vi "Meas Result Get Sweep Data.vi"(3 "freq filter (NaN: no filter)":dbl=nan, 4 "uncertainty mode":T1, 5 "phase index (default: 0)":i32, 6 "result":T4) -> (0 "quantities":T2, 1 "unc(data)":T3, 2 "data":T3)   [LabVIEW 2013]
doc: "Processes collected readings into sweep with uncertainties in selected mode."
uses:
  Meas Results Sweep Data.ctl
  Meas Results.ctl
  bridge/Bridge Frequency Readings Data.ctl
  drivers/TWM client/Meas Proc QWTB Spectrum Data.ctl
  Meas Quantity Names.ctl
  Meas Results Sweep Data Uncertainty Mode.ctl
  varilib/varilib.lvlib
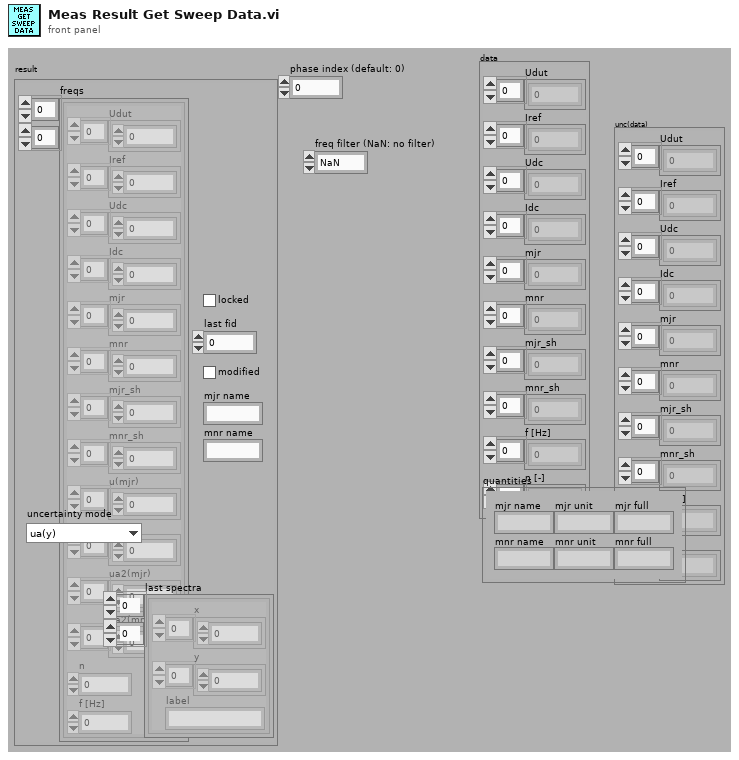
[diagram p1: front panel]
types:
  T1 = typedef "Meas Results Sweep Data Uncertainty Mode.ctl" = enum16{"ua(y)", "ua(y) (p=95%)", "uc(y) (p=95%)"}
  T2 = typedef "Meas Quantity Names.ctl" = cluster{"mjr name":string, "mnr name":string, "mjr unit":string, "mnr unit":string, "mjr full":string, "mnr full":string}
  T3 = typedef "Meas Results Sweep Data.ctl" = cluster{"Udut":dbl[], "Iref":dbl[], "Udc":dbl[], "Idc":dbl[], "mjr":dbl[], "mnr":dbl[], "mjr_sh":dbl[], "mnr_sh":dbl[], "f [Hz]":dbl[], "n [-]":i32[]}
  T4 = typedef "Meas Results.ctl" = cluster{"freqs":T5[][], "locked":bool, "last fid":i32, "modified":bool, "mjr name":string, "mnr name":string, "last spectra":T6[][]}
  T5 = typedef "Bridge Frequency Readings Data.ctl" = cluster{"Udut":dbl[], "Iref":dbl[], "Udc":dbl[], "Idc":dbl[], "mjr":dbl[], "mnr":dbl[], "mjr_sh":dbl[], "mnr_sh":dbl[], "u(mjr)":dbl[], "u(mnr)":dbl[], "ua2(mjr)":dbl[], "ua2(mnr)":dbl[], "n":i32, "f [Hz]":dbl}
  T6 = typedef "Meas Proc QWTB Spectrum Data.ctl" = cluster{"x":sgl[], "y":sgl[], "label":string}
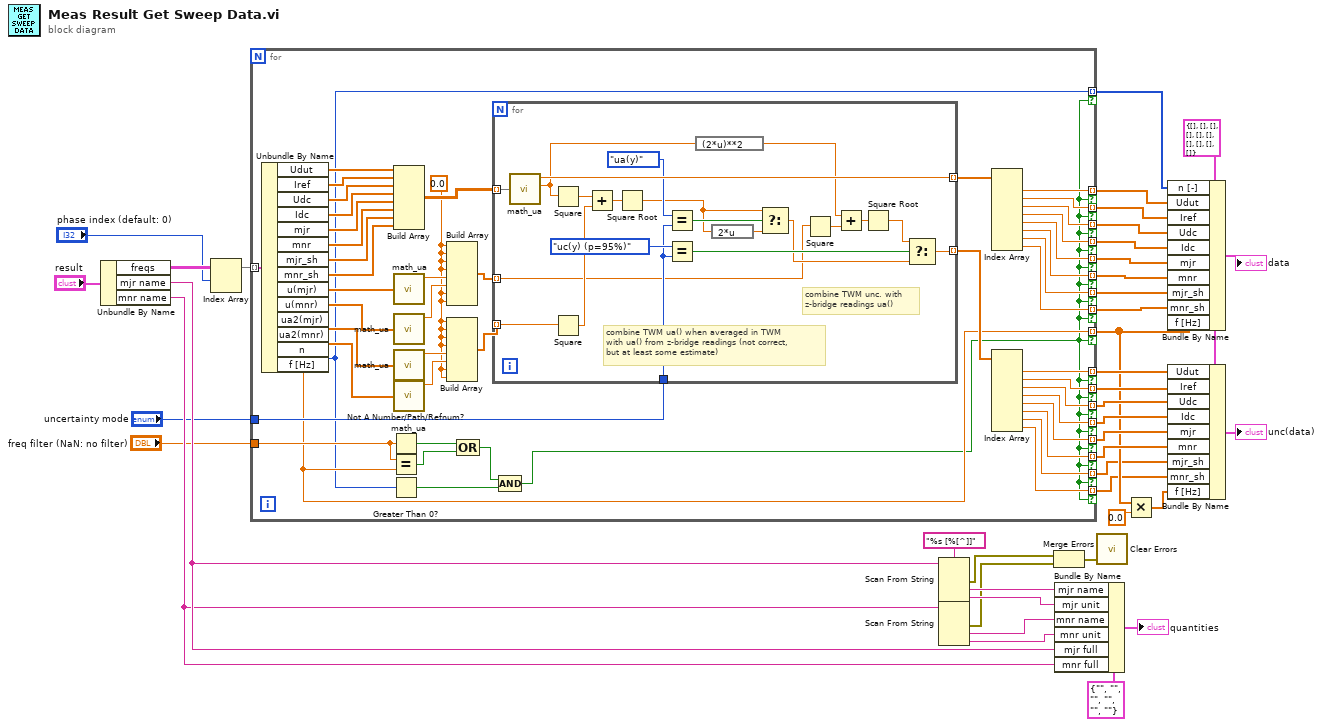
[diagram p0: block diagram]
diagram:
  w18 = "%s [%[^]]" ("format string")
  w24 = T3 {"Udut"=[], "Iref"=[], "Udc"=[], "Idc"=[], "mjr"=[], "mnr"=[], "mjr_sh"=[], "mnr_sh"=[], "f [Hz]"=[], "n [-]"=[]} ("data")
  n1 = Unbundle By Name("result") -> ("freqs"=w40:T5[][], "mjr name"=w15:string, "mnr name"=w14:string)
  n2 = Index Array(array=w40, index (row)="phase index (default: 0)") -> (element=w4:T5[])  [unwired: 1 in]
  n3 = for {
    tunnel: w4 -> [w89] mode=indexing
    tunnel: [w80] -> w39 mode=indexing if=w42
    tunnel: [w79] -> w38 mode=indexing if=w42
    tunnel: [w78] -> w37 mode=indexing if=w42
    tunnel: [w77] -> w36 mode=indexing if=w42
    tunnel: [w76] -> w35 mode=indexing if=w42
    tunnel: [w75] -> w34 mode=indexing if=w42
    tunnel: [w48] -> w26 mode=indexing if=w42
    tunnel: [w73] -> w33 mode=indexing if=w42
    tunnel: [w72] -> w32 mode=indexing if=w42
    tunnel: [w71] -> w31 mode=indexing if=w42
    tunnel: [w70] -> w30 mode=indexing if=w42
    tunnel: [w69] -> w29 mode=indexing if=w42
    tunnel: [w68] -> w28 mode=indexing if=w42
    tunnel: "uncertainty mode" -> [w57]
    tunnel: [w54] -> w8 mode=indexing if=w42
    tunnel: [w53] -> w7 mode=indexing if=w42
    tunnel: [w52] -> w6 mode=indexing if=w42
    tunnel: [w51] -> w5 mode=indexing if=w42
    tunnel: "freq filter (NaN: no filter)" -> [w49]
    tunnel: [w43] -> w1 mode=indexing if=w42
    w50 = 0.0
    n4 = Unbundle By Name(w89) -> ("Udut"=w88:dbl[], "Iref"=w87:dbl[], "Udc"=w86:dbl[], "Idc"=w85:dbl[], "mjr"=w84:dbl[], "mnr"=w83:dbl[], "mjr_sh"=w56:dbl[], "mnr_sh"=w55:dbl[], "u(mjr)"=w67:dbl[], "u(mnr)"=w66:dbl[], "ua2(mjr)"=w65:dbl[], "ua2(mnr)"=w64:dbl[], "n"=w43:i32, "f [Hz]"=w48:dbl)
    n5 = Not A Number/Path/Refnum?(number/path/refnum=w49) -> (NaN/Path/Refnum?=w47:bool)
    n6 = Equal?(x=w49, y=w48) -> (x = y?=w46:bool)
    n7 = Greater Than 0?(x=w43) -> (x > 0?=w45:bool)
    n8 = Build Array(w88, w87, w86, w85, w84, w83, w56, w55) -> (w82:dbl[][])
    n9 = call "math_ua.vi"("x"=w67) -> ("mean(x)"=w63:dbl)  [unwired: 3 out]
    n10 = call "math_ua.vi"("x"=w66) -> ("mean(x)"=w62:dbl)  [unwired: 3 out]
    n11 = call "math_ua.vi"("x"=w65) -> ("mean(x)"=w61:dbl)  [unwired: 3 out]
    n12 = call "math_ua.vi"("x"=w64) -> ("mean(x)"=w60:dbl)  [unwired: 3 out]
    n13 = Build Array(w50, w50, w50, w50, w63, w62, w50, w50) -> (w59:dbl[])
    n14 = Build Array(w50, w50, w50, w50, w61, w60, w50, w50) -> (w58:dbl[])
    n15 = Compound Arithmetic op=OR(w47, w46) -> (w44:bool)
    n16 = for {
      tunnel: w82 -> [w90] mode=indexing
      tunnel: [w110] -> w81 mode=indexing
      tunnel: [w97] -> w74 mode=indexing
      tunnel: w59 -> [w95] mode=indexing
      tunnel: w58 -> [w109] mode=indexing
      tunnel: w57 -> [w102]
      # "combine TWM ua() when averaged in TWM\nwith ua() from z-bridge readings (not correct,\nbut at least some estimate)"
      # "combine TWM unc. with\nz-bridge readings ua()"
      n17 = call "math_ua.vi"("x"=w90) -> ("mean(x)"=w110:dbl, "ua(x)"=w96:dbl)  [unwired: 2 out]
      n18 = Square(x=w96) -> (x^2=w108:dbl)
      n19 = Square(x=w109) -> (x^2=w107:dbl)
      n20 = Add(x=w108, y=w107) -> (x+y=w106:dbl)
      n21 = Square Root(x=w106) -> (sqrt(x)=w99:dbl)
      n22 = Equal?(x=Meas_Results_Sweep_Data_Uncertainty_Mode."ua(y)", y=w102) -> (x = y?=w103:bool)
      n23 = Equal?(x=Meas_Results_Sweep_Data_Uncertainty_Mode."uc(y) (p=95%)", y=w102) -> (x = y?=w105:bool)
      n24 = expression code="(2*u)**2"(w96) -> (w93:dbl)
      n25 = expression code="2*u"(w99) -> (w98:dbl)
      n26 = Select(t=w99, s=w103, f=w98) -> (s? t:f=w100:dbl)
      n27 = Square(x=w95) -> (x^2=w94:dbl)
      n28 = Add(x=w93, y=w94) -> (x+y=w92:dbl)
      n29 = Square Root(x=w92) -> (sqrt(x)=w91:dbl)
      n30 = Select(t=w91, s=w105, f=w100) -> (s? t:f=w97:dbl)
    }
    n31 = Compound Arithmetic op=AND(w44, w45) -> (w42:bool)
    n32 = Index Array(array=w81) -> (element #1=w80:dbl, element #2=w79:dbl, element #3=w78:dbl, element #4=w77:dbl, element #5=w76:dbl, element #6=w75:dbl, element #7=w54:dbl, element #8=w53:dbl)  [unwired: 8 in]
    n33 = Index Array(array=w74) -> (element #1=w73:dbl, element #2=w72:dbl, element #3=w71:dbl, element #4=w70:dbl, element #5=w69:dbl, element #6=w68:dbl, element #7=w52:dbl, element #8=w51:dbl)  [unwired: 8 in]
  }
  n34 = Scan From String(format string=w18, input string=w15) -> (error out=w11:errorcluster, output 1=w20:string, output 2=w19:string)  [unwired: 4 in, 2 out]
  n35 = Scan From String(format string=w18, input string=w14) -> (error out=w12:errorcluster, output 1=w17:string, output 2=w16:string)  [unwired: 4 in, 2 out]
  n36 = Merge Errors(w11, w12) -> (w10:errorcluster)
  n37 = Bundle By Name(cluster=T2 {"mjr name"="", "mnr name"="", "mjr unit"="", "mnr unit"="", "mjr full"="", "mnr full"=""} ("quantities"), "mjr name"=w20, "mjr unit"=w19, "mnr name"=w17, "mnr unit"=w16, "mjr full"=w15, "mnr full"=w14) -> (→"quantities":T2)
  n38 = call <vilib>:"Clear Errors.vi"("error in (no error)"=w10) -> ()  [unwired: 6 in, 1 out]
  n39 = Multiply(x=w26, y=0.0) -> (x*y=w27:dbl[])
  n40 = Bundle By Name(cluster=w24, "n [-]"=w1, "Udut"=w39, "Iref"=w38, "Udc"=w37, "Idc"=w36, "mjr"=w35, "mnr"=w34, "mjr_sh"=w8, "mnr_sh"=w7, "f [Hz]"=w26) -> (→"data":T3)
  n41 = Bundle By Name(cluster=w24, "Udut"=w33, "Iref"=w32, "Udc"=w31, "Idc"=w30, "mjr"=w29, "mnr"=w28, "mjr_sh"=w6, "mnr_sh"=w5, "f [Hz]"=w27) -> (→"unc(data)":T3)
